vi "Parse XML.vi"(8 "Error In":errorcluster, 11 "XML String Input":string) -> (0 "Error Out":errorcluster, 3 "Parsed Value":string)   [LabVIEW 2022 SP3, in "MU_3SL_interface.lvlib"]
uses:
  MU_3SL_interface.lvlib
  <vilib>/regexp/Match Regular Expression.xnode
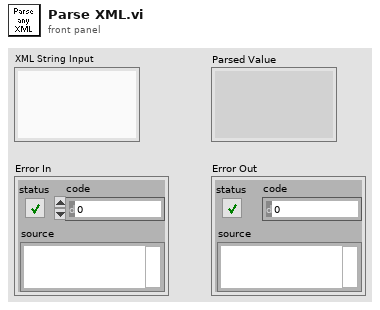
[diagram p1: front panel]
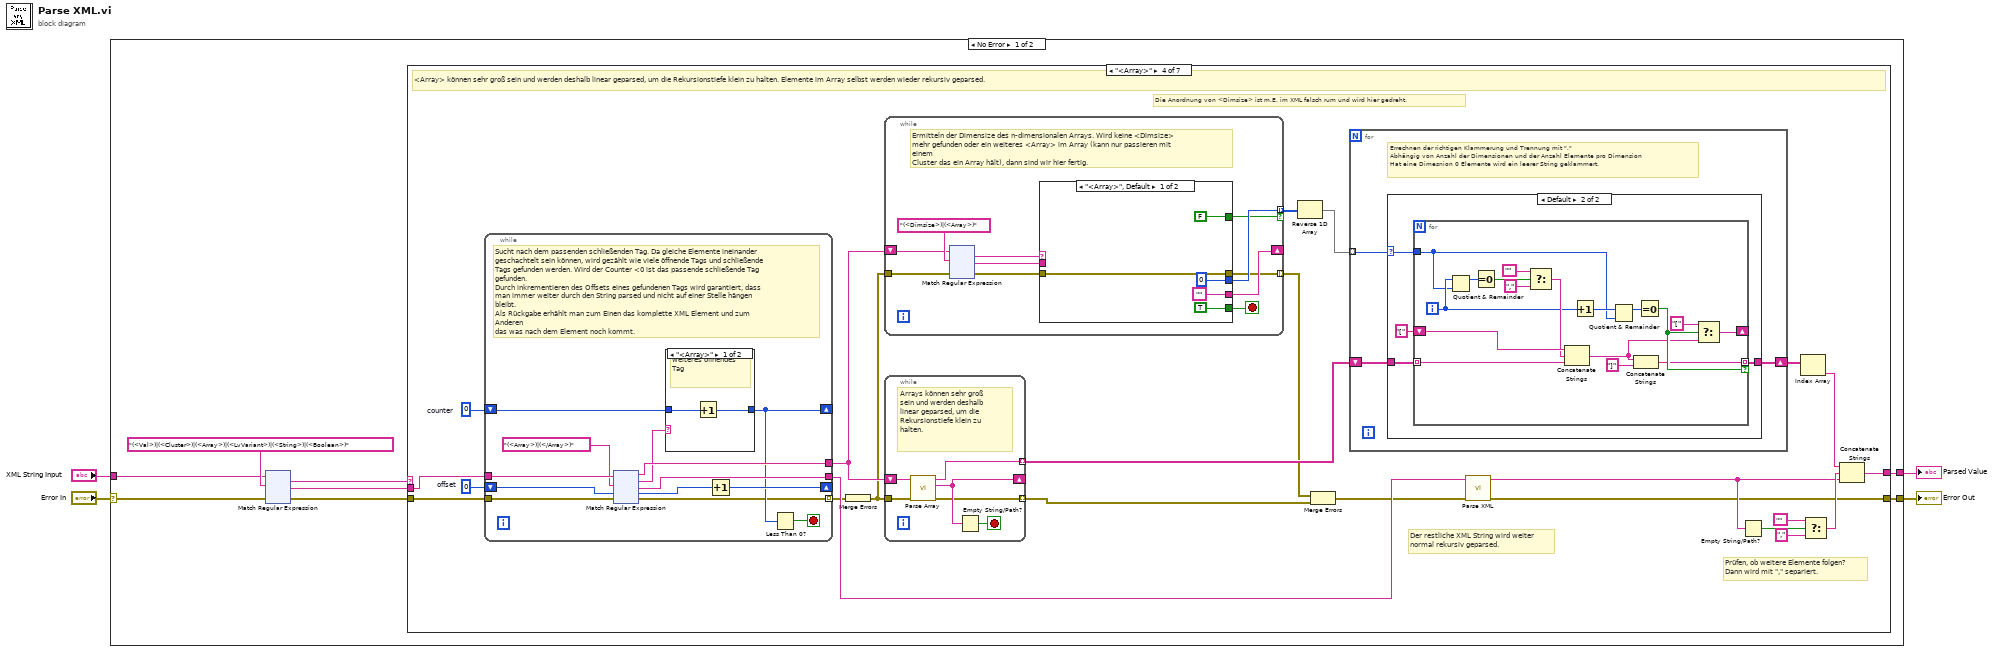
[diagram p0: block diagram]
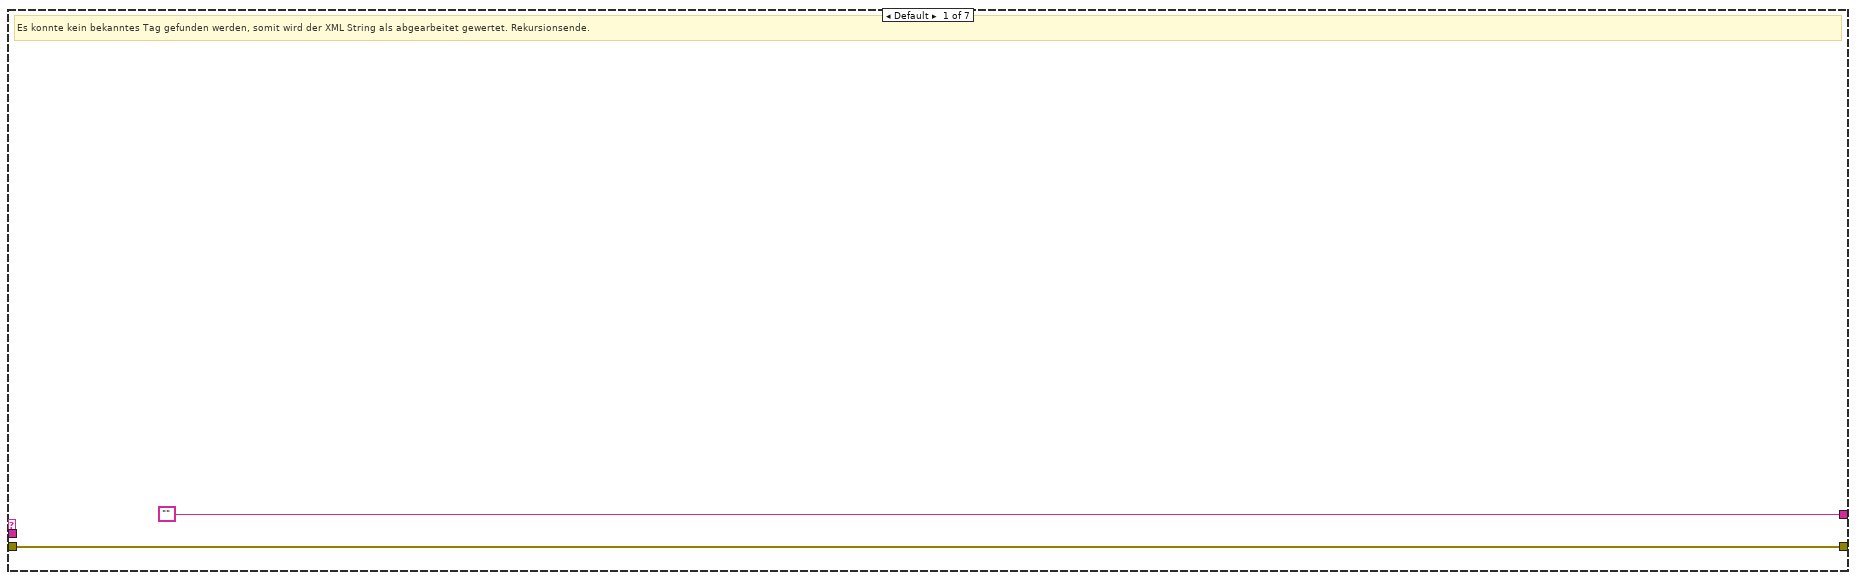
[diagram p2: hidden frame]
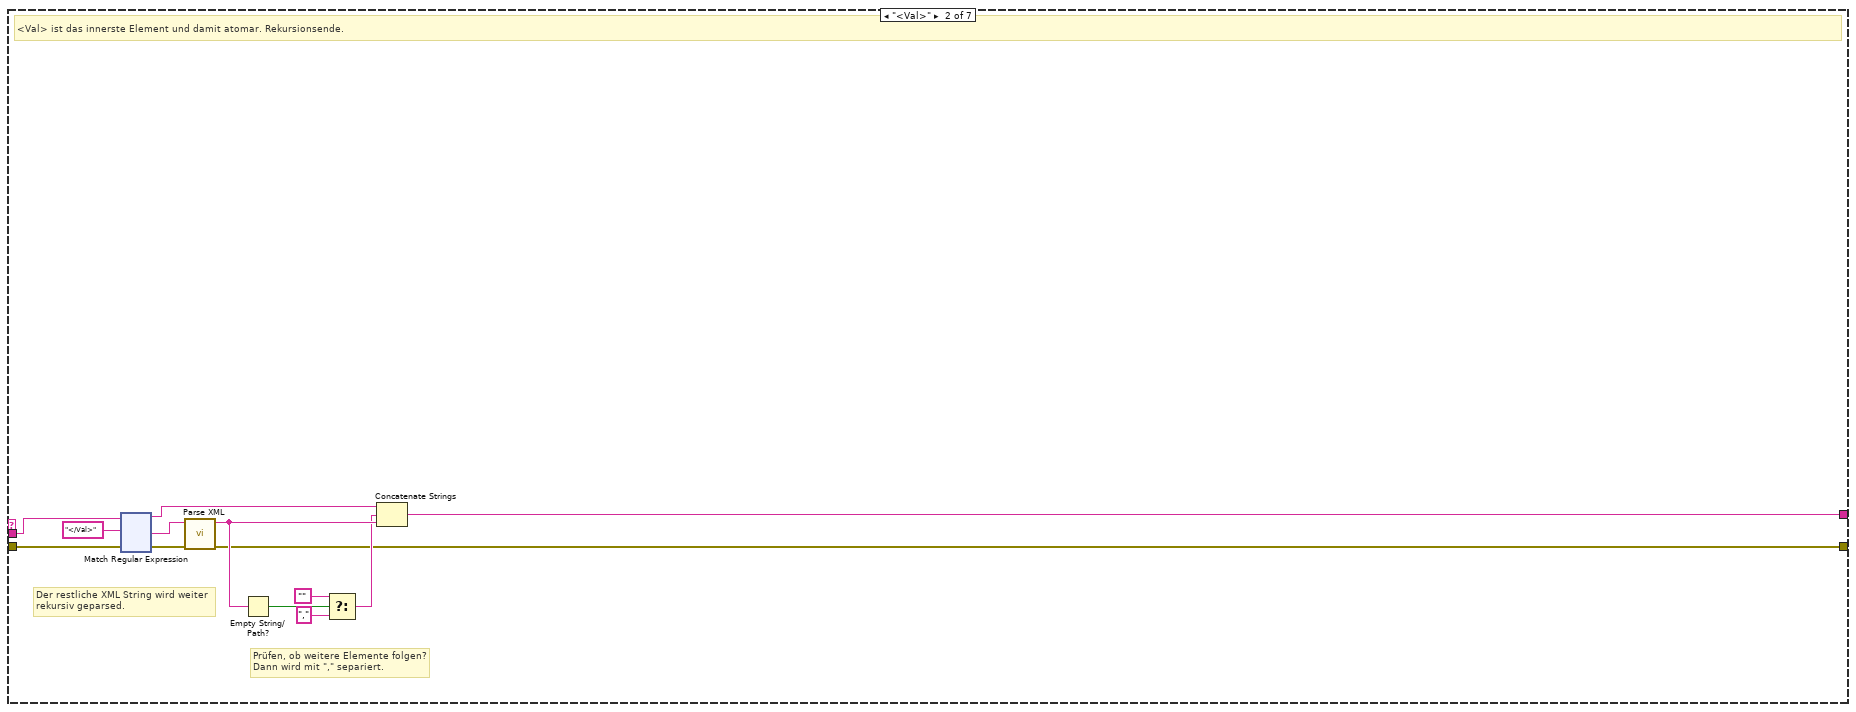
[diagram p3: hidden frame]
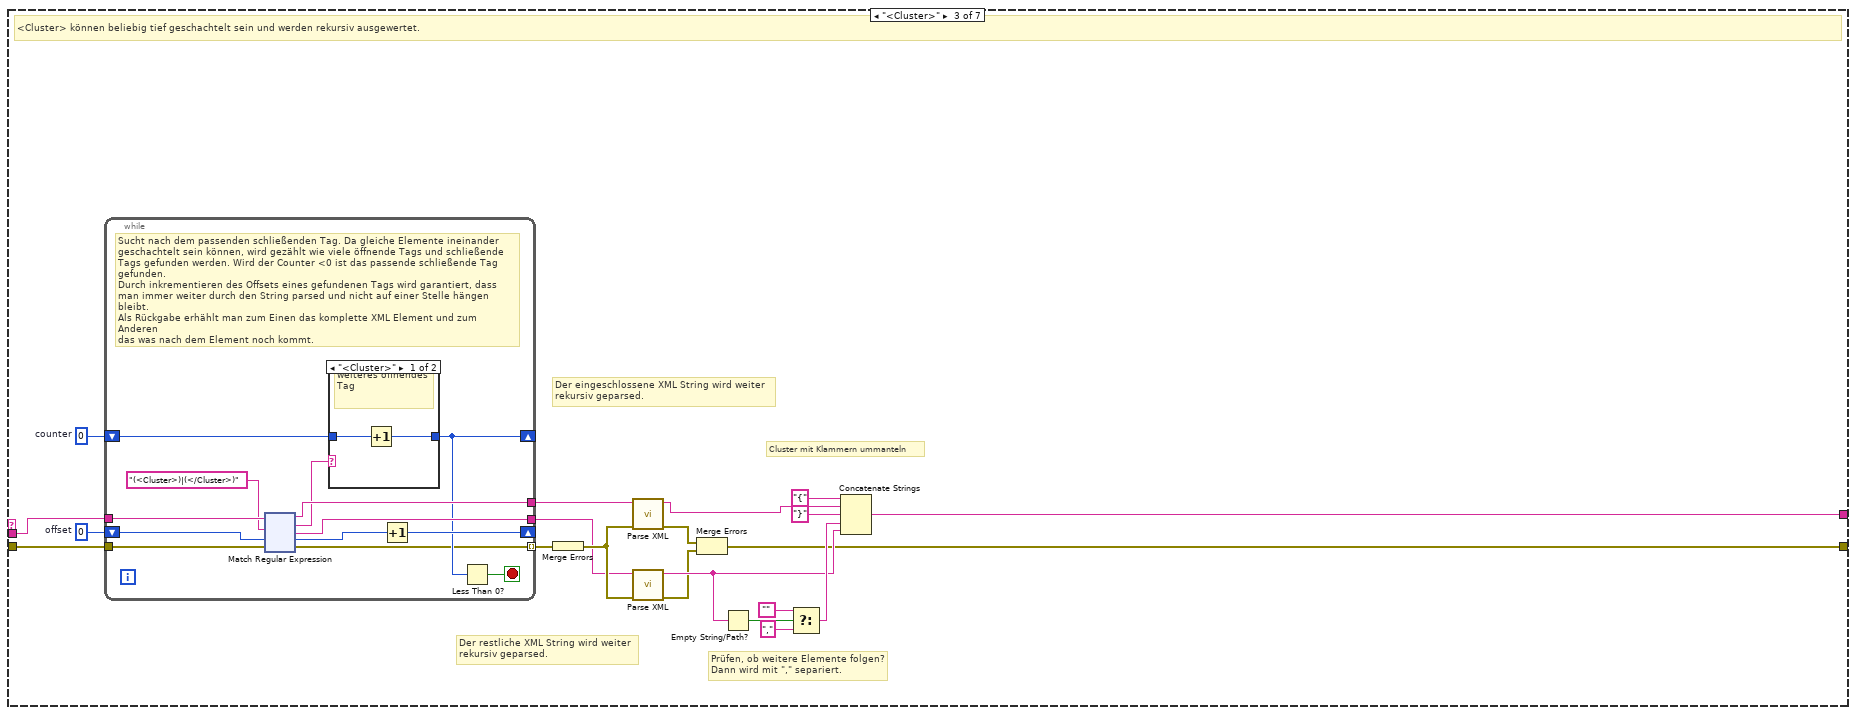
[diagram p4: hidden frame]
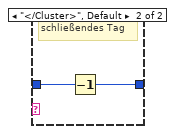
[diagram p5: hidden frame]
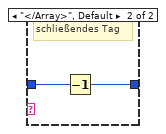
[diagram p6: hidden frame]
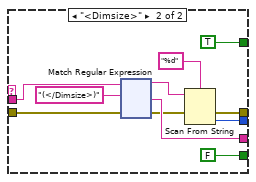
[diagram p7: hidden frame]
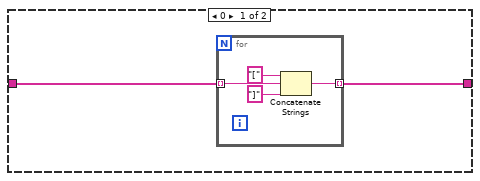
[diagram p8: hidden frame]
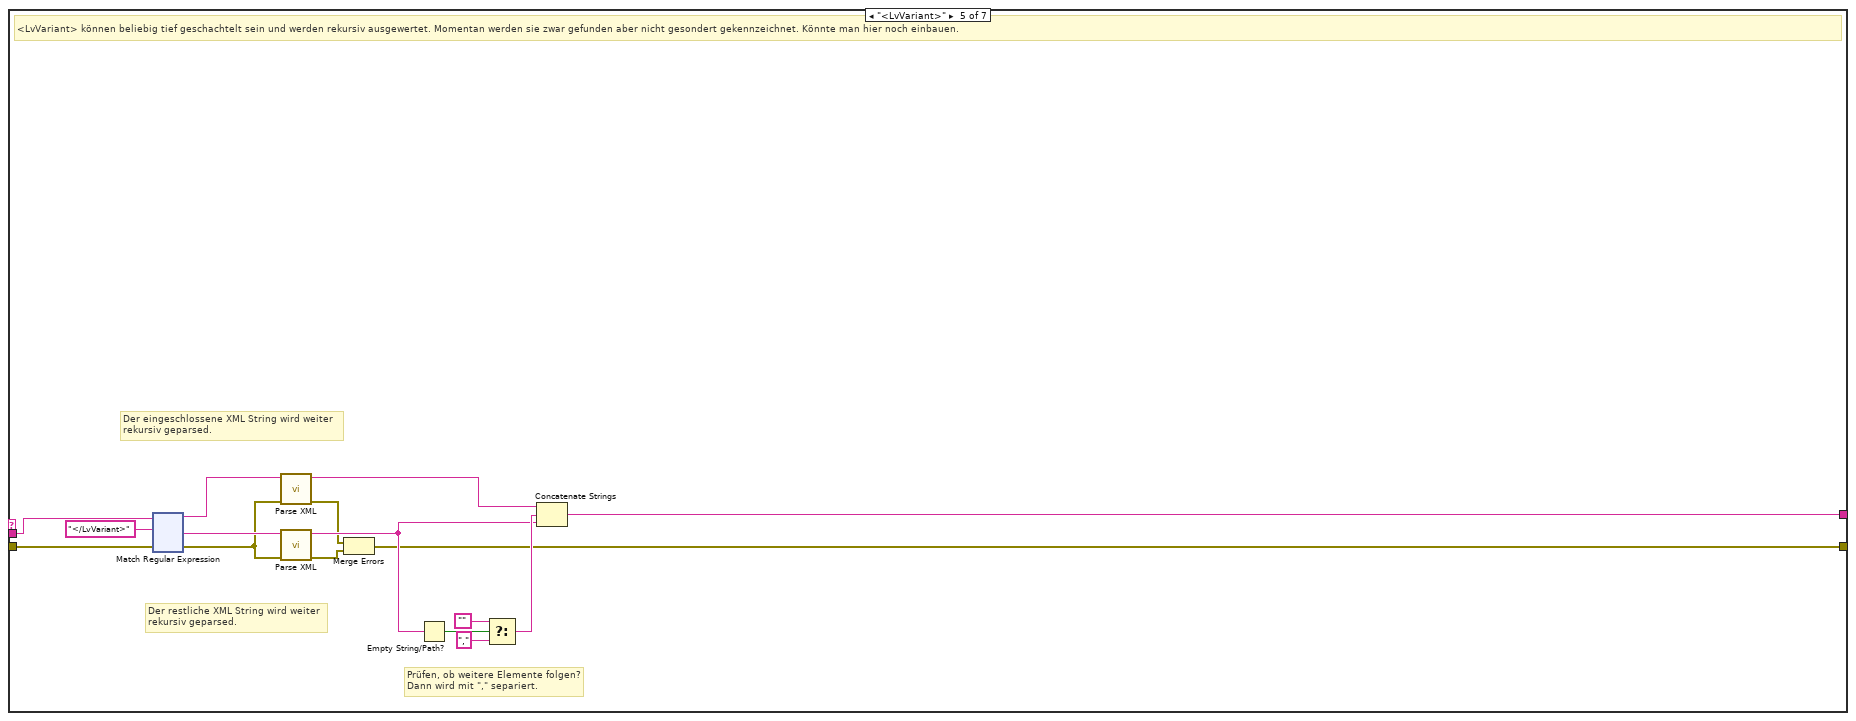
[diagram p9: hidden frame]
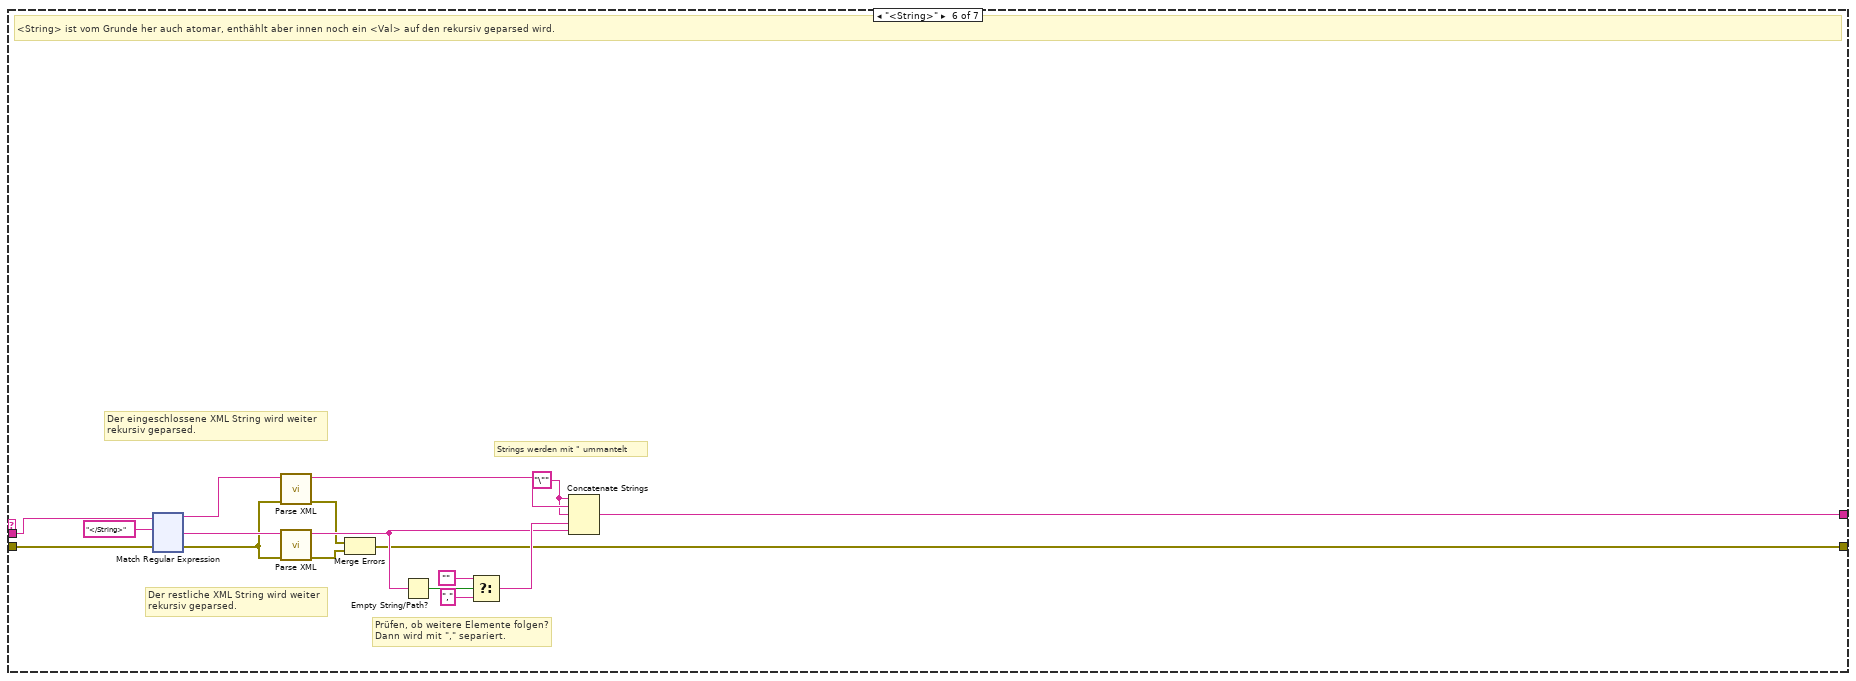
[diagram p10: hidden frame]
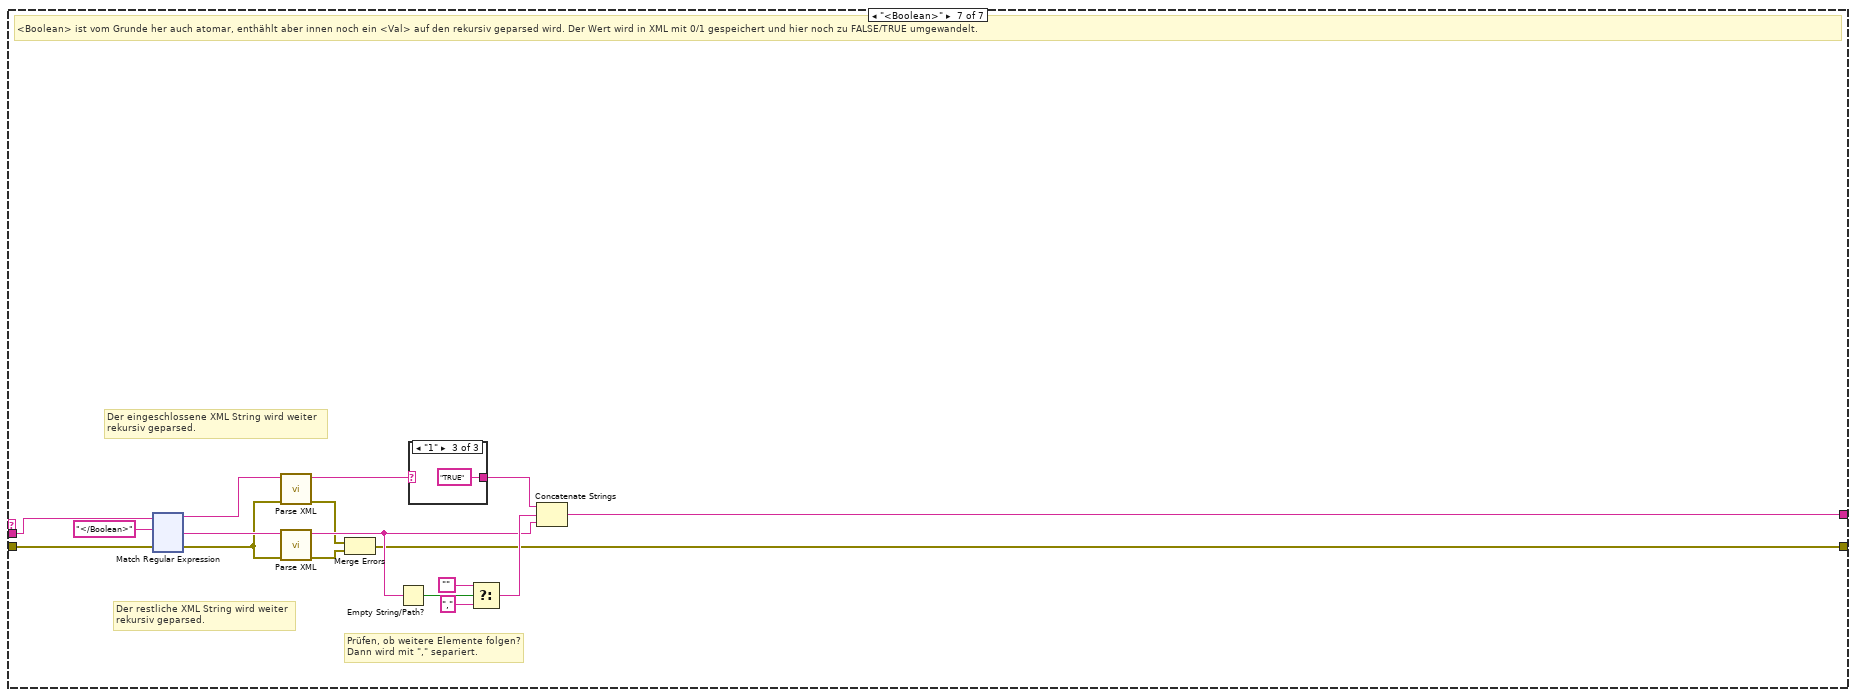
[diagram p11: hidden frame]
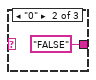
[diagram p13: hidden frame]
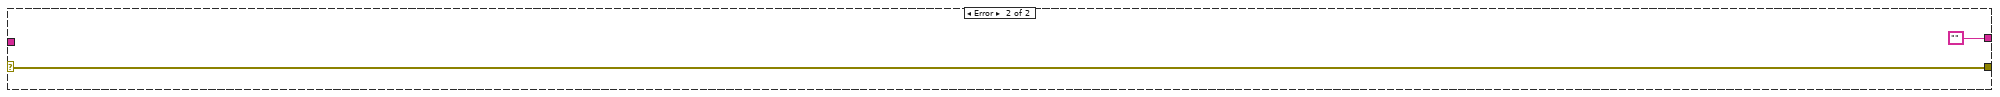
[diagram p14: hidden frame]
diagram:
  n1 = case shown="No Error" "Error In" {
    selector: "Error In" -> [w7 w1275]
    tunnel: [w9 ""] -> w4
    tunnel: "XML String Input" -> [w8 _]
    tunnel: [w5 w1275] -> w1
    frame No Error {
      n2 = xnode "Match Regular Expression"("input string"=w8, "regular expression"="(<Val>)|(<Cluster>)|(<Array>)|(<LvVariant>)|(<String>)|(<Boolean>)", "error in"=w7) -> ("whole match"=w11:string, "after match"=w10:string, "error out"=w6:errorcluster)  [unwired: 3 in, 2 out]
      n3 = case shown="\"<Array>\"" w11 {
        tunnel: ["" ("regular expression") w24 w164 w321 w766 w900 w1034] -> w9
        tunnel: w10 -> [_ w26 w152 w309 w765 w899 w1033]
        tunnel: w6 -> [w13 w17 w155 w310 w757 w891 w1024]
        tunnel: [w13 w15 w145 w302 w753 w886 w1020] -> w5
        frame Default {
          # "Es konnte kein bekanntes Tag gefunden werden, somit wird der XML String als abgearbeitet gewertet. Rekursionsende."
        }
        frame "<Val>" {
          # "Prüfen, ob weitere Elemente folgen?\nDann wird mit \",\" separiert."
          # "Der restliche XML String wird weiter \nrekursiv geparsed."
          # "<Val> ist das innerste Element und damit atomar. Rekursionsende."
          n4 = xnode "Match Regular Expression"("input string"=w26, "regular expression"="</Val>", "error in"=w17) -> ("before match"=w18:string, "after match"=w25:string, "error out"=w16:errorcluster)  [unwired: 3 in, 2 out]
          n5 = call "Parse XML.vi"("Error In"=w16, "XML String Input"=w25) -> ("Error Out"=w15:errorcluster, "Parsed Value"=w23:string)  [unwired: 8 in]
          n6 = Empty String/Path?(string/path=w23) -> (empty?=w22:bool)
          n7 = Select(t="", s=w22, f="," ("string")) -> (s? t:f=w19:string)
          n8 = Concatenate Strings(w18, w19, w23) -> (w24:string)
        }
        frame "<Cluster>" {
          w153 = 0  # offset
          w154 = 0  # counter
          # "Cluster mit Klammern ummanteln"
          # "Prüfen, ob weitere Elemente folgen?\nDann wird mit \",\" separiert."
          # "Der restliche XML String wird weiter \nrekursiv geparsed."
          # "Der eingeschlossene XML String wird weiter \nrekursiv geparsed."
          # "<Cluster> können beliebig tief geschachtelt sein und werden rekursiv ausgewertet."
          n9 = while {
            tunnel: [w174] -> w149
            shift-right: [w170] -> _
            shift-left: w153 -> [w172]
            shift-right: [w168] -> _
            shift-left: w154 -> [w169]
            tunnel: w152 -> [w177]
            tunnel: [w175] -> w148
            tunnel: w155 -> [w166]
            tunnel: [w165] -> w151 mode=indexing
            stop <- w167 stop-if-true
            # "Sucht nach dem passenden schließenden Tag. Da gleiche Elemente ineinander\ngeschachtelt sein können, wird gezählt wie viele öffnende Tags und schließende\nTags gefunden werden. Wird der Counter <0 ist das passende schließende Tag\ngefunden.\nDurch inkrementieren des Offsets eines gefundenen Tags wird garantiert, dass \nman immer weiter durch den String parsed und nicht auf einer Stelle hängen bleibt.\nAls Rückgabe erhählt man zum Einen das komplette XML Element und zum Anderen\ndas was nach dem Element noch kommt."
            n10 = xnode "Match Regular Expression"("input string"=w177, "regular expression"="(<Cluster>)|(</Cluster>)", "offset (0)"=w172, "error in"=w166) -> ("before match"=w175:string, "whole match"=w173:string, "after match"=w174:string, "offset past match"=w171:i32, "error out"=w165:errorcluster)  [unwired: 2 in]
            n11 = case shown="\"<Cluster>\"" w173 {
              tunnel: w169 -> [w179 w181]
              tunnel: [w178 w180] -> w168
              frame "<Cluster>" {
                # "weiteres öffnendes Tag"
                n12 = Increment(x=w179) -> (x+1=w178:i32)
              }
              frame "</Cluster>", Default {
                # "schließendes Tag"
                n13 = Decrement(x=w181) -> (x-1=w180:i32)
              }
            }
            n14 = Increment(x=w171) -> (x+1=w170:i32)
            n15 = Less Than 0?(x=w168) -> (x < 0?=w167:bool)
          }
          n16 = Merge Errors(w151) -> (w150:errorcluster)
          n17 = call "Parse XML.vi"("Error In"=w150, "XML String Input"=w148) -> ("Error Out"=w146:errorcluster, "Parsed Value"=w156:string)  [unwired: 8 in]
          n18 = call "Parse XML.vi"("Error In"=w150, "XML String Input"=w149) -> ("Error Out"=w147:errorcluster, "Parsed Value"=w158:string)  [unwired: 8 in]
          n19 = Merge Errors(w146, w147) -> (w145:errorcluster)
          n20 = Empty String/Path?(string/path=w158) -> (empty?=w161:bool)
          n21 = Select(t="", s=w161, f="," ("string")) -> (s? t:f=w159:string)
          n22 = Concatenate Strings("{" ("string"), w156, "}" ("string"), w159, w158) -> (w164:string)
        }
        frame "<Array>" {
          w308 = 0  # counter
          w307 = 0  # offset
          # "Prüfen, ob weitere Elemente folgen?\nDann wird mit \",\" separiert."
          # "Die Anordnung von <Dimsize> ist m.E. im XML falsch rum und wird hier gedreht."
          # "Der restliche XML String wird weiter \nnormal rekursiv geparsed."
          # "<Array> können sehr groß sein und werden deshalb linear geparsed, um die Rekursionstiefe klein zu halten. Elemente im Array selbst werden wieder rekursiv geparsed."
          n23 = while {
            tunnel: [w337] -> w306
            shift-right: [w333] -> _
            shift-left: w307 -> [w335]
            shift-right: [w331] -> _
            shift-left: w308 -> [w332]
            tunnel: w309 -> [w340]
            tunnel: [w338] -> w301
            tunnel: w310 -> [w329]
            tunnel: [w328] -> w305 mode=indexing
            stop <- w330 stop-if-true
            # "Sucht nach dem passenden schließenden Tag. Da gleiche Elemente ineinander\ngeschachtelt sein können, wird gezählt wie viele öffnende Tags und schließende\nTags gefunden werden. Wird der Counter <0 ist das passende schließende Tag\ngefunden.\nDurch inkrementieren des Offsets eines gefundenen Tags wird garantiert, dass \nman immer weiter durch den String parsed und nicht auf einer Stelle hängen bleibt.\nAls Rückgabe erhählt man zum Einen das komplette XML Element und zum Anderen\ndas was nach dem Element noch kommt."
            n24 = xnode "Match Regular Expression"("input string"=w340, "regular expression"="(<Array>)|(</Array>)", "offset (0)"=w335, "error in"=w329) -> ("before match"=w338:string, "whole match"=w336:string, "after match"=w337:string, "offset past match"=w334:i32, "error out"=w328:errorcluster)  [unwired: 2 in]
            n25 = case shown="\"<Array>\"" w336 {
              tunnel: w332 -> [w342 w344]
              tunnel: [w341 w343] -> w331
              frame "<Array>" {
                # "weiteres öffnendes Tag"
                n26 = Increment(x=w342) -> (x+1=w341:i32)
              }
              frame "</Array>", Default {
                # "schließendes Tag"
                n27 = Decrement(x=w344) -> (x-1=w343:i32)
              }
            }
            n28 = Increment(x=w334) -> (x+1=w333:i32)
            n29 = Less Than 0?(x=w331) -> (x < 0?=w330:bool)
          }
          n30 = Merge Errors(w305) -> (w300:errorcluster)
          n31 = while {
            shift-right: [w470] -> _
            shift-left: w301 -> [w471]
            tunnel: [w468] -> w312 mode=indexing if=w466
            tunnel: w300 -> [w464]
            tunnel: [w462] -> w304 mode=indexing
            stop <- w469 stop-if-true
            # "Ermitteln der Dimensize des n-dimensionalen Arrays. Wird keine <Dimsize> mehr gefunden oder ein weiteres <Array> im Array (kann nur passieren mit einem\nCluster das ein Array hält), dann sind wir hier fertig."
            n32 = xnode "Match Regular Expression"("input string"=w471, "regular expression"="(<Dimsize>)|(<Array>)", "error in"=w464) -> ("whole match"=w465:string, "after match"=w467:string, "error out"=w463:errorcluster)  [unwired: 3 in, 2 out]
            n33 = case shown="\"<Array>\", Default" w465 {
              tunnel: ["" w484] -> w470
              tunnel: [TRUE FALSE] -> w469
              tunnel: [0 w488] -> w468
              tunnel: w467 -> [_ w487]
              tunnel: [FALSE TRUE] -> w466
              tunnel: w463 -> [w473 w483]
              tunnel: [w473 w478] -> w462
              frame "<Array>", Default {
              }
              frame "<Dimsize>" {
                n34 = xnode "Match Regular Expression"("input string"=w487, "regular expression"="(</Dimsize>)", "error in"=w483) -> ("before match"=w485:string, "after match"=w484:string, "error out"=w481:errorcluster)  [unwired: 3 in, 2 out]
                n35 = Scan From String(format string="%d", input string=w485, error in=w481) -> (error out=w478:errorcluster, output 1=w488:i32)  [unwired: 2 in, 2 out]
              }
            }
          }
          n36 = while {
            shift-right: [w326] -> _
            shift-left: w301 -> [w327]
            tunnel: [w324] -> w315 mode=indexing
            tunnel: w300 -> [w323]
            tunnel: [w322] -> w299 mode=indexing
            stop <- w325 stop-if-true
            # "Arrays können sehr groß sein und werden deshalb linear geparsed, um die Rekursionstiefe klein zu halten."
            n37 = call "Parse Array.vi"("Error In"=w323, "Array XML String Input"=w327) -> ("Error Out"=w322:errorcluster, "Rest String"=w326:string, "Array Val"=w324:string)  [unwired: 7 in]
            n38 = Empty String/Path?(string/path=w326) -> (empty?=w325:bool)
          }
          n39 = Reverse 1D Array(array=w312) -> (reversed array=w311:i32[])
          n40 = Merge Errors(w304, w299) -> (w303:errorcluster)
          n41 = for {
            tunnel: w311 -> [w724] mode=indexing
            shift-right: [w723] -> w314
            shift-left: w315 -> [w725]
            # "Errechnen der richtigen Klammerung und Trennung mit \",\"\nAbhängig von Anzahl der Dimensionen und der Anzahl Elemente pro Dimension\nHat eine Dimesnion 0 Elemente wird ein leerer String geklammert."
            n42 = case shown="Default" w724 {
              selector: w724 -> [_ w734]
              tunnel: w725 -> [w727 w735]
              tunnel: [w726 w732] -> w723
              frame 0 {
                n43 = for {
                  tunnel: w727 -> [w729] mode=indexing
                  tunnel: [w728] -> w726 mode=indexing
                  n44 = Concatenate Strings("[" ("string"), w729, "]" ("string")) -> (w728:string)
                }
              }
              frame Default {
                n45 = for {
                  tunnel: w735 -> [w749] mode=indexing
                  tunnel: w734 -> [w737]
                  shift-right: [w747] -> _
                  shift-left: "[" -> [w750]
                  tunnel: [w739] -> w732 mode=indexing if=w748
                  i -> [w738]
                  n46 = Quotient & Remainder(x=w738, y=w737) -> (x-y*floor(x/y)=w736:i32)  [unwired: 1 out]
                  n47 = Equal To 0?(x=w736) -> (x = 0?=w745:bool)
                  n48 = Select(t="" ("string"), s=w745, f="," ("string")) -> (s? t:f=w742:string)
                  n49 = Concatenate Strings(w750, w742, w749) -> (w741:string)
                  n50 = Increment(x=w738) -> (x+1=w751:i32)
                  n51 = Quotient & Remainder(x=w751, y=w737) -> (x-y*floor(x/y)=w752:i32)  [unwired: 1 out]
                  n52 = Concatenate Strings(w741, "]") -> (w739:string)
                  n53 = Equal To 0?(x=w752) -> (x = 0?=w748:bool)
                  n54 = Select(t="[", s=w748, f=w741) -> (s? t:f=w747:string)
                }
              }
            }
          }
          n55 = call "Parse XML.vi"("Error In"=w303, "XML String Input"=w306) -> ("Error Out"=w302:errorcluster, "Parsed Value"=w316:string)  [unwired: 8 in]
          n56 = Empty String/Path?(string/path=w316) -> (empty?=w320:bool)
          n57 = Index Array(array=w314) -> (element=w313:string)  [unwired: 1 in]
          n58 = Select(t="", s=w320, f="," ("string")) -> (s? t:f=w317:string)
          n59 = Concatenate Strings(w313, w317, w316) -> (w321:string)
        }
        frame "<LvVariant>" {
          # "Prüfen, ob weitere Elemente folgen?\nDann wird mit \",\" separiert."
          # "Der eingeschlossene XML String wird weiter \nrekursiv geparsed."
          # "Der restliche XML String wird weiter \nrekursiv geparsed."
          # "<LvVariant> können beliebig tief geschachtelt sein und werden rekursiv ausgewertet. Momentan werden sie zwar gefunden aber nicht gesondert gekennzeichnet. Könnte man hier noch einbauen."
          n60 = xnode "Match Regular Expression"("input string"=w765, "regular expression"="</LvVariant>", "error in"=w757) -> ("before match"=w768:string, "after match"=w767:string, "error out"=w756:errorcluster)  [unwired: 3 in, 2 out]
          n61 = call "Parse XML.vi"("Error In"=w756, "XML String Input"=w768) -> ("Error Out"=w754:errorcluster, "Parsed Value"=w758:string)  [unwired: 8 in]
          n62 = call "Parse XML.vi"("Error In"=w756, "XML String Input"=w767) -> ("Error Out"=w755:errorcluster, "Parsed Value"=w759:string)  [unwired: 8 in]
          n63 = Merge Errors(w754, w755) -> (w753:errorcluster)
          n64 = Empty String/Path?(string/path=w759) -> (empty?=w763:bool)
          n65 = Select(t="", s=w763, f="," ("string")) -> (s? t:f=w760:string)
          n66 = Concatenate Strings(w758, w760, w759) -> (w766:string)
        }
        frame "<String>" {
          w887 = "\"" ("string")
          # "Strings werden mit \" ummantelt"
          # "Prüfen, ob weitere Elemente folgen?\nDann wird mit \",\" separiert."
          # "Der restliche XML String wird weiter \nrekursiv geparsed."
          # "Der eingeschlossene XML String wird weiter \nrekursiv geparsed."
          # "<String> ist vom Grunde her auch atomar, enthählt aber innen noch ein <Val> auf den rekursiv geparsed wird."
          n67 = xnode "Match Regular Expression"("input string"=w899, "regular expression"="</String>", "error in"=w891) -> ("before match"=w902:string, "after match"=w901:string, "error out"=w890:errorcluster)  [unwired: 3 in, 2 out]
          n68 = call "Parse XML.vi"("Error In"=w890, "XML String Input"=w902) -> ("Error Out"=w888:errorcluster, "Parsed Value"=w892:string)  [unwired: 8 in]
          n69 = call "Parse XML.vi"("Error In"=w890, "XML String Input"=w901) -> ("Error Out"=w889:errorcluster, "Parsed Value"=w893:string)  [unwired: 8 in]
          n70 = Merge Errors(w888, w889) -> (w886:errorcluster)
          n71 = Empty String/Path?(string/path=w893) -> (empty?=w897:bool)
          n72 = Select(t="", s=w897, f="," ("string")) -> (s? t:f=w894:string)
          n73 = Concatenate Strings(w887, w892, w887, w894, w893) -> (w900:string)
        }
        frame "<Boolean>" {
          # "Prüfen, ob weitere Elemente folgen?\nDann wird mit \",\" separiert."
          # "Der restliche XML String wird weiter \nrekursiv geparsed."
          # "Der eingeschlossene XML String wird weiter \nrekursiv geparsed."
          # "<Boolean> ist vom Grunde her auch atomar, enthählt aber innen noch ein <Val> auf den rekursiv geparsed wird. Der Wert wird in XML mit 0/1 gespeichert und hier noch zu FALSE/TRUE umgewandelt."
          n74 = xnode "Match Regular Expression"("input string"=w1033, "regular expression"="</Boolean>", "error in"=w1024) -> ("before match"=w1036:string, "after match"=w1035:string, "error out"=w1022:errorcluster)  [unwired: 3 in, 2 out]
          n75 = call "Parse XML.vi"("Error In"=w1022, "XML String Input"=w1036) -> ("Error Out"=w1023:errorcluster, "Parsed Value"=w1026:string)  [unwired: 8 in]
          n76 = call "Parse XML.vi"("Error In"=w1022, "XML String Input"=w1035) -> ("Error Out"=w1021:errorcluster, "Parsed Value"=w1027:string)  [unwired: 8 in]
          n77 = Merge Errors(w1023, w1021) -> (w1020:errorcluster)
          n78 = Empty String/Path?(string/path=w1027) -> (empty?=w1031:bool)
          n79 = case shown="\"1\"" w1026 {
            selector: w1026 -> [w1037 _ _]
            tunnel: [w1037 "FALSE" ("string") "TRUE" ("string")] -> w1025
            frame Default {
            }
            frame "0" {
            }
            frame "1" {
            }
          }
          n80 = Select(t="", s=w1031, f="," ("string")) -> (s? t:f=w1028:string)
          n81 = Concatenate Strings(w1025, w1028, w1027) -> (w1034:string)
        }
      }
    }
    frame Error {
    }
  }
  "Parsed Value" <- w4
  "Error Out" <- w1
